vi "Write I64 Direct.vi"(8 "error in (no error)":errorcluster, 9 "Timeout (ms)":i32, 10 "Data":i64, 11 "CIFTag in":refnum<class "CIF_CIPC_Chn_I64.lvclass">) -> (0 "error out":errorcluster, 1 "timed out?":bool, 3 "CIFTag out":refnum<class "CIF_CIPC_Chn_I64.lvclass">)   [LabVIEW 2021, in "CIF_CIPC_Chn_I64.lvclass"]
uses:
  CIF_CIPC_Chn_I64.lvclass
  D:/dev/Packages/CIF_Channels_Core/src/CIFChannels/CIFChannels.lvclass
  D:/dev/Packages/CIF_Channels_Core/src/CIPC_Channels/CIF_CIPC_Chan/CIF_CIPC_Chn.lvclass
  CIFChannels/CIFChannels.lvclass/CIFChannels.ctl
  CIF_CIPC_Chan/CIF_CIPC_Chn.lvclass/CIF_CIPC_Chn.ctl
  CIF_CIPC_Chn_I64.lvclass/CIF_CIPC_Chn_I64.ctl
  4dec1408-e4ff-48ac-a735-b713bf84484a.vi
  CIFChannels/Accessors/Read Tag Forced.vi
  <vilib>/CIF Foundation/CIF CIPC/SubVIs/Check Error.vi
  <vilib>/CIF Foundation/CIF CIPC/SubVIs/Get Element Write Position.vi
  <vilib>/CIF Foundation/CIF CIPC/SubVIs/Notify Of New Write.vi
  <vilib>/CIF Foundation/CIF CIPC/SubVIs/Get dll Path.vi
  <vilib>/CIF Foundation/CIF CIPC/SubVIs/Get Element Info Variant.vi
  <vilib>/Utility/error.llb/Trim Whitespace.vi
  <vilib>/Utility/error.llb/Error Cluster From Error Code.vi
  CIF_CIPC_Chan/CIF_CIPC_Chn.lvclass
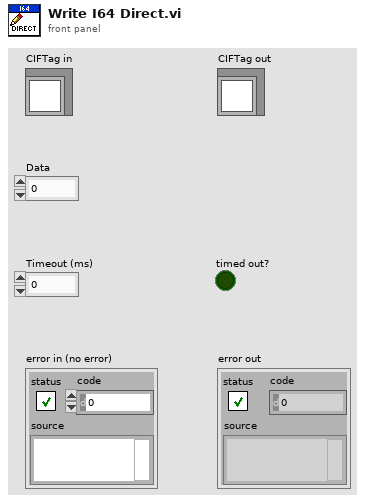
[diagram p1: front panel]
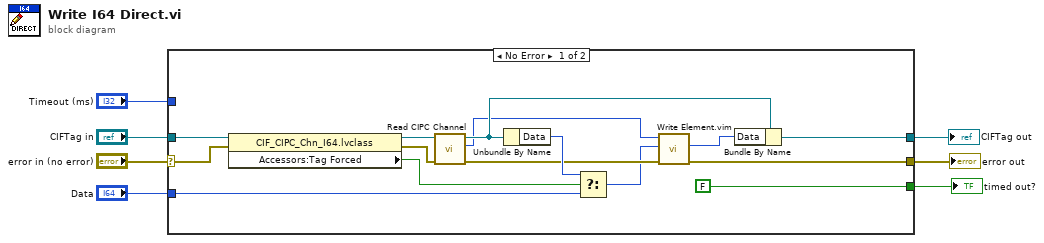
[diagram p0: block diagram]
diagram:
  n1 = case shown="No Error" "error in (no error)" {
    selector: "error in (no error)" -> [w21 w24]
    tunnel: [w10 w24] -> w2
    tunnel: [w11 w23] -> w3
    tunnel: "CIFTag in" -> [w22 w23]
    tunnel: "Data" -> [w19 _]
    tunnel: [FALSE ("Timed out?") _] -> w1
    tunnel: "Timeout (ms)" -> [_ _]
    frame No Error {
      n2 = property class="CIF_CIPC_Chn_I64.lvclass"(reference=w22, error in=w21) -> (reference out=w17:refnum<class "CIF_CIPC_Chn_I64.lvclass">, error out=w16:errorcluster, "Accessors:Tag Forced"=w20:bool)
      n3 = call "Read CIPC Channel.vi"("error in (no error)"=w16, "CIFTag in"=w17) -> ("error out"=w14:errorcluster, "CIF Channel"=w13:u64, "CIFTag out"=w15:refnum<class "CIF_CIPC_Chn_I64.lvclass">)  [unwired: 7 in]
      n4 = Unbundle By Name(w15) -> ("Data"=w18:i64)
      n5 = Select(t=w18, s=w20, f=w19) -> (s? t:f=w12:i64)
      n6 = call "Write Element.vim"("error in (no error)"=w14, "Data in"=w12, "CIPC Reference in"=w13) -> ("error out"=w10:errorcluster, "Data out"=w9:i64)  [unwired: 5 in, 2 out]
      n7 = Bundle By Name(cluster=w15, "Data"=w9) -> (w11:refnum<class "CIF_CIPC_Chn_I64.lvclass">)
    }
    frame Error {
    }
  }
  "error out" <- w2
  "CIFTag out" <- w3
  "timed out?" <- w1
